vi "UpdateEmptyCase.vi"(10 "test":T1(array[cluster])) -> (2 "test 2":T1(array[cluster]))   [LabVIEW 2018, in "Sequences.lvlib"]
uses:
  Sequences.lvlib
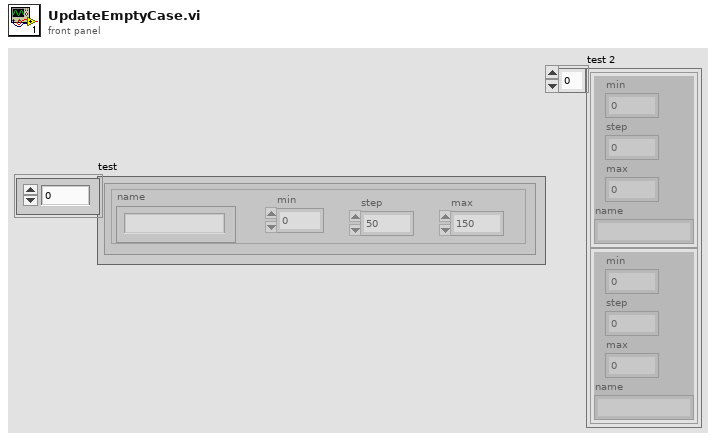
[diagram p1: front panel]
types:
  T1 = cluster{"min":dbl, "step":dbl, "max":dbl, "name":string}[]
  T2 = cluster{"min":dbl, "step":dbl, "max":dbl, "name":string}
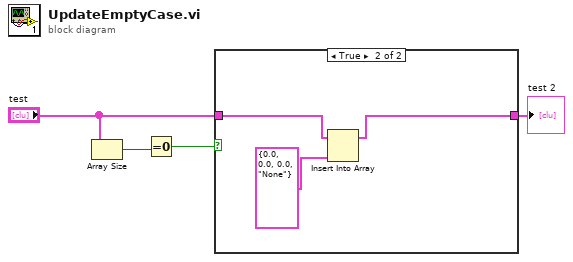
[diagram p0: block diagram]
diagram:
  n1 = Array Size(array="test") -> (size(s)=w4:i32)
  n2 = Equal To 0?(x=w4) -> (x = 0?=w3:bool)
  n3 = case shown="True" w3 {
    tunnel: "test" -> [w5 w8]
    tunnel: [w5 w6] -> w1
    frame False {
    }
    frame True {
      n4 = Insert Into Array(array=w8, new element=T2 {"min"=0.0, "step"=0.0, "max"=0.0, "name"="None"} ("new element/subarray")) -> (w6:T1)  [unwired: 1 in]
    }
  }
  "test 2" <- w1
